vi "Trackit.vi"(8 "error out":errorcluster) -> (0 "error out 2":errorcluster, 1 "Frame tracked":i32)   [LabVIEW 2011, in "OfflineTracker.lvlib"]
uses:
  OfflineTracker.lvlib
  <vilib>/Utility/file.llb/Read From Spreadsheet File (DBL).vi
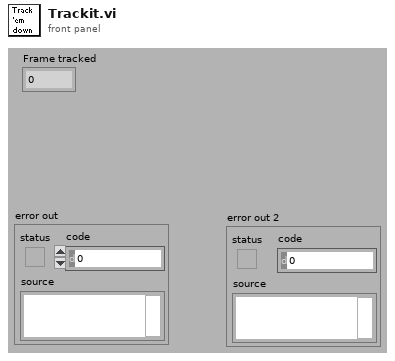
[diagram p1: front panel]
types:
  T1 = enum16{"init", "get", "set single frame", "set all"}
  T2 = typedef "IMAQ Image.ctl" = refnum<image>
  T3 = cluster{"front panel settings":cluster{"files":cluster{"LUT path":path, "Trace path":path, " folders #":i32, "base path":path, "use trace":bool, "use base":bool, "LUT tmp":i32, "Trace tmp":i32, "active path":path}, "Tracking":cluster{"RminZ (pix)":i32, "Rmax (pix)":i32, "angular pixel \ncoverage factor":dbl, "radial pixel \ncoverage factor":dbl}, "Frames":cluster{"Start frame":i32, "number of frames":u32, "display frame ":i32, "track every nd frame ":i32, "Track all frames":bool, "active frame":i32}, "Calibs":cluster{"Zlut number of steps":i32, "pix/um":dbl, "Z correction factor":dbl, "Zlut step size (um)":dbl, "ROI(pix)":i32}, "Beads":cluster{"number of ref beads":i32, "overlay":bool}, "Misc":cluster{"save images to new location":bool, "destination":path}}, "data":cluster{"Image":T2, "image size":i32[], "Bead Array":i32[][], "overlay image":T2, "# beads":i32, "Job list":string[][], "job running":bool, "job #":i32, "folders to go":i32}}
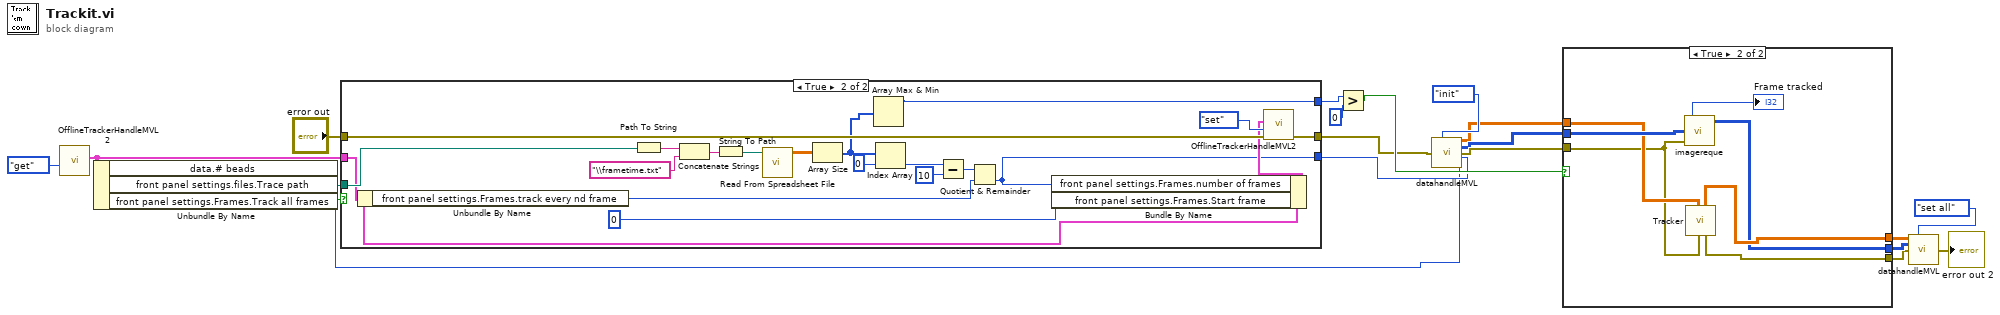
[diagram p0: block diagram]
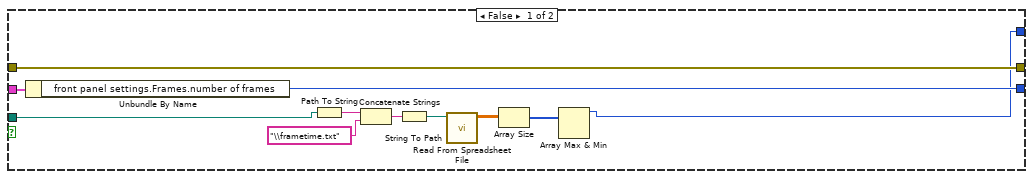
[diagram p3: hidden frame]
diagram:
  n1 = call "OfflineTrackerHandleMVL2.vi"("action"=enum16{"get", "set"}."get") -> ("out"=w18:T3)  [unwired: 5 in, 1 out]
  n2 = Unbundle By Name(w18) -> ("data.# beads"=w11:i32, "front panel settings.files.Trace path"=w19:path, "front panel settings.Frames.Track all frames"=w16:bool)
  n3 = case shown="True" w16 {
    tunnel: [w31 w34] -> w12
    tunnel: w18 -> [w30 w36]
    tunnel: w19 -> [w23 w46]
    tunnel: [w29 w38] -> w9
    tunnel: "error out" -> [w29 w37]
    tunnel: [w21 w32] -> w15
    frame False {
      n4 = Unbundle By Name(w30) -> ("front panel settings.Frames.number of frames"=w31:u32)
      n5 = Path To String(path=w23) -> (string=w28:string)
      n6 = Concatenate Strings(w28, "\\frametime.txt" ("string")) -> (w26:string)
      n7 = String To Path(string=w26) -> (path=w27:path)
      n8 = call-poly <vilib>:"Read From Spreadsheet File.vi"("file path (dialog if empty)"=w27) -> ("all rows"=w24:dbl[][])  [unwired: 3 in, 7 out]
      n9 = Array Size(array=w24) -> (size(s)=w22:i32[])
      n10 = Array Max & Min(array=w22) -> (max value=w21:i32)  [unwired: 3 out]
    }
    frame True {
      n11 = Unbundle By Name(w36) -> ("front panel settings.Frames.track every nd frame"=w43:i32)
      n12 = Path To String(path=w46) -> (string=w50:string)
      n13 = Concatenate Strings(w50, "\\frametime.txt" ("string")) -> (w48:string)
      n14 = String To Path(string=w48) -> (path=w49:path)
      n15 = call-poly <vilib>:"Read From Spreadsheet File.vi"("file path (dialog if empty)"=w49) -> ("all rows"=w45:dbl[][])  [unwired: 3 in, 7 out]
      n16 = Array Size(array=w45) -> (size(s)=w33:i32[])
      n17 = Array Max & Min(array=w33) -> (max value=w32:i32)  [unwired: 3 out]
      n18 = Index Array(array=w33, index=0) -> (element=w42:i32)
      n19 = Subtract(x=w42, y=10) -> (x-y=w41:i32)
      n20 = Quotient & Remainder(x=w41, y=w43) -> (floor(x/y)=w34:i32)  [unwired: 1 out]
      n21 = Bundle By Name(cluster=w36, "front panel settings.Frames.number of frames"=w34, "front panel settings.Frames.Start frame"=0 ("Start frame")) -> (w35:T3)
      n22 = call "OfflineTrackerHandleMVL2.vi"("error in"=w37, "action"=enum16{"get", "set"}."set", "in"=w35) -> ("error out"=w38:errorcluster)  [unwired: 3 in, 1 out]
    }
  }
  n23 = Greater?(x=w15, y=0) -> (0:w13:bool)
  n24 = call "datahandleMVL.vi"("action"=T1."init", "error in"=w9, "number of frames"=w12, "number of beads"=w11) -> ("XYZ out"=w6:dbl[][][], "time out"=w7:i32[][], "error in 2"=w8:errorcluster)  [unwired: 6 in, 3 out]
  n25 = case shown="True" w13 {
    tunnel: w8 -> [w52 w58]
    tunnel: w7 -> [w53 w60]
    tunnel: w6 -> [w54 w59]
    tunnel: [w54 w57] -> w3
    tunnel: [w53 w56] -> w2
    tunnel: [w52 w55] -> w1
    frame False {
    }
    frame True {
      n26 = call "imagereque.vi"("error in"=w58, "Time data in"=w60) -> ("Time data out"=w56:i32[][], "Frame"=→"Frame tracked":i32)  [unwired: 1 in, 1 out]
      n27 = call "Tracker.vi"("error in"=w58, "XYZdata in"=w59) -> ("error in 2"=w55:errorcluster, "XYZdata out"=w57:dbl[][][])  [unwired: 7 in, 1 out]
    }
  }
  n28 = call "datahandleMVL.vi"("xyz array in"=w3, "action"=T1."set all", "Time array in"=w2, "error in"=w1) -> ("error in 2"=→"error out 2":errorcluster)  [unwired: 6 in, 5 out]
